vi "Msg Create UI Message Queue.vi"(5 "Event Registration Refnum in":refnum<event-registration>, 6 "error in (no error)":errorcluster) -> (0 "error out":errorcluster, 3 "user event":refnum<user-event>, 4 "Event Registration Refnum out":refnum<event-registration>)   [LabVIEW 2014]
doc: "Create a \"message queue\" that enables posting of events to an event structure. \n\nThis is part of the Msg suite, intended to make messaging architectures in LabVIEW\nSee the template \"Message Based Application Template.vi\" for normal usage.\n\nCopyright 2005-2016 Jason Sommerville\n\nThis VI may be freely used, modified or distributed under the BSD license."
uses:
  Message Cluster.ctl
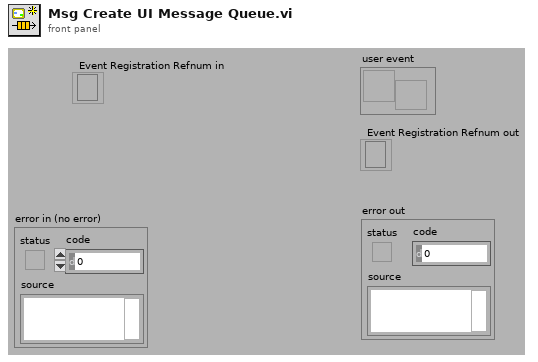
[diagram p1: front panel]
types:
  T1 = typedef "Message Cluster.ctl" = cluster{"Message":string, "Data":variant, "Response Notifier":refnum<notifier>}
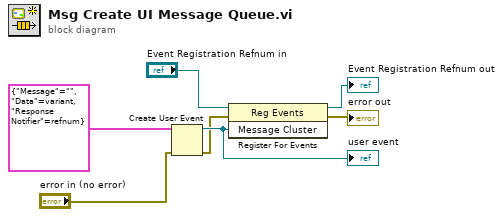
[diagram p0: block diagram]
diagram:
  n1 = Create User Event(user event datatype=T1 {"Message"="", "Data"=variant, "Response Notifier"=refnum} ("Message Cluster"), error in="error in (no error)") -> (user event=w5:refnum<user-event>, error out=w4:errorcluster)
  "user event" <- w5
  n2 = register-events(reference="Event Registration Refnum in", error in=w4, w5) -> (reference out=→"Event Registration Refnum out":refnum<event-registration>, error out=→"error out":errorcluster)
